vi "ip_change_wp.vi"() -> ()   [LabVIEW 2022 SP3]
uses:
  <vilib>/addons/database/Connection.llb/DB Tools Open Connec (String).vi
  <vilib>/addons/database/NI_Database_API.lvlib
panel:
  in  "OK Button":bool
  out "error out 2":errorcluster
  in  "error in (no error) 2":errorcluster
  in  "new_IP":string
  in  "intrface_name":string(combo)
  in  "stop":bool
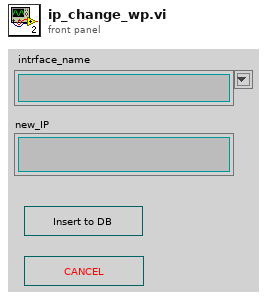
[diagram p1: front panel]
types:
  T1 = typedef "NI_Database_API.lvlib/Conn ObjectReference.ctl" = refnum<k1>
  T2 = cluster{" intrface_name":string, "new_IP ":string}
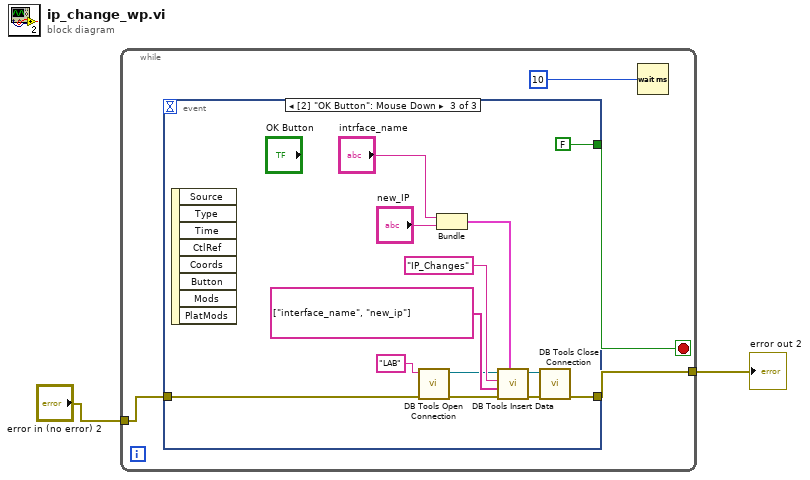
[diagram p0: block diagram]
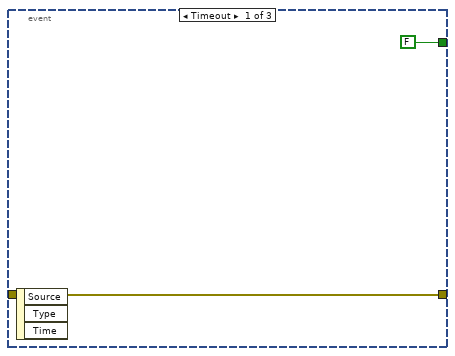
[diagram p2: hidden frame]
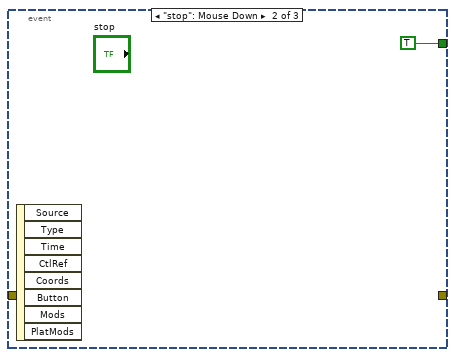
[diagram p3: hidden frame]
diagram:
  n1 = while {
    tunnel: "error in (no error) 2" -> [w4]
    tunnel: [w3] -> w1
    stop <- w6 stop-if-true
    n2 = event shown="[2] \"OK Button\": Mouse Down" {
      selector: _ -> [_ _ _]
      dyn-events: _ -> [_ _ _]
      timeout: _ -> [_ _ _]
      tunnel: [FALSE TRUE FALSE] -> w6
      tunnel: w4 -> [w7 _ w11]
      tunnel: [w7 _ w10] -> w3
      event Timeout {
        n3 = event-data() -> ()  [unwired: 1 in, 3 out]
      }
      event "stop": Mouse Down {
        n4 = event-data() -> ()  [unwired: 1 in, 8 out]
      }
      event "OK Button": Mouse Down {
        n5 = event-data() -> ()  [unwired: 1 in, 8 out]
        n6 = call-poly <vilib>:"DB Tools Open Connection.vi"("error in (no error)"=w11, "connection information"="LAB") -> ("error out"=w16:errorcluster, "connection reference"=w17:T1)  [unwired: 6 in]
        n7 = Bundle("intrface_name"="intrface_name", "new_IP"="new_IP") -> (w13:T2)  [unwired: 1 in]
        n8 = call <vilib>:"DB Tools Insert Data.vi"("data"=w13, "error in (no error)"=w16, "columns"=string[] ["interface_name", "new_ip"], "table"="IP_Changes", "connection reference"=w17) -> ("error out"=w18:errorcluster, "connection reference out"=w19:T1)  [unwired: 5 in]
        n9 = call <vilib>:"DB Tools Close Connection.vi"("error in (no error)"=w18, "connection reference"=w19) -> ("error out"=w10:errorcluster)  [unwired: 5 in]
      }
    }
    n10 = Wait (ms)(milliseconds to wait=u32 10) -> ()  [unwired: 1 out]
  }
  "error out 2" <- w1
